vi "DAC Configure FP View.vi"(8 "error in":errorcluster, 11 "DAC TC Temperature in":refnum<class "DAC TC Temperature.lvclass">) -> (0 "error out":errorcluster, 3 "DAC TC Temperature out":refnum<class "DAC TC Temperature.lvclass">)   [LabVIEW 2019, in "DAC.lvlib" / "DAC TC Temperature.lvclass"]
uses:
  DAC TC Temperature.lvclass
  C:/Users/wg/Documents/LV_Projects/test-stand/App/DAC/DAC.lvclass
  Results/Results Method.ctl
  Results/DeepU Results/DeepU Results.lvclass
  DAC.lvclass/DAC.ctl
  DAC TC Temperature.lvclass/DAC TC Temperature.ctl
  Results/Results.lvlib
  DAC.lvclass
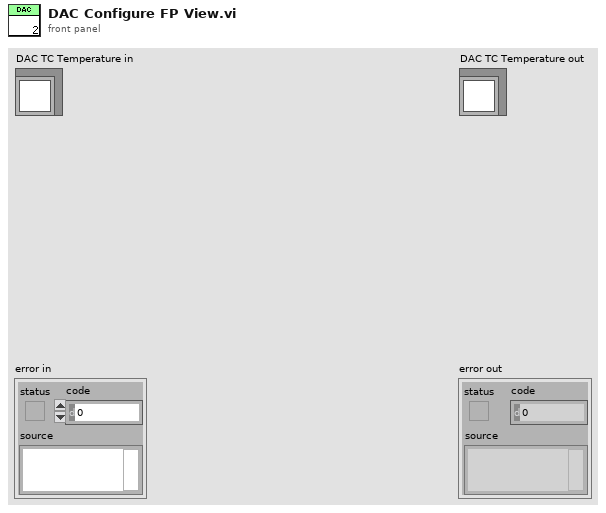
[diagram p1: front panel]
types:
  T1 = typedef "Results.lvlib/Results Method.ctl" = enum16{"Get", "Set"}
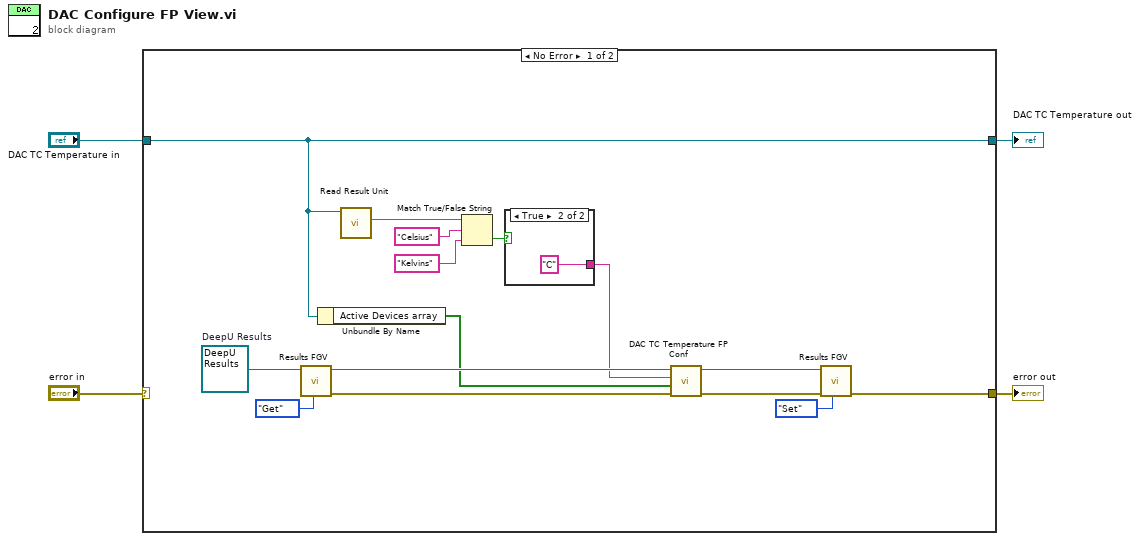
[diagram p0: block diagram]
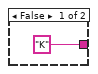
[diagram p2: hidden frame]
diagram:
  n1 = case shown="No Error" "error in" {
    selector: "error in" -> [_ w23]
    tunnel: [w19 w23] -> w1
    tunnel: [w11 w22] -> w2
    tunnel: "DAC TC Temperature in" -> [w11 w22]
    frame No Error {
      w18 = refnum<class "DeepU Results.lvclass"> refnum  # DeepU Results
      n2 = call-dynamic "Results FGV.vi"("Method"=Results_Method."Get", "DeepU Results in"=w18) -> ("error out"=w13:errorcluster, "DeepU Results out"=w15:refnum<class "DeepU Results.lvclass">)  [unwired: 8 in]
      n3 = Unbundle By Name(w11) -> ("Active Devices array"=w10:bool[])
      n4 = call "Read Result Unit.vi"("DAC in"=w11) -> ("Unit"=w6:string)  [unwired: 8 in, 2 out]
      n5 = Match True/False String(2:"Kelvins" ("false string"), 3:"Celsius" ("true string"), 4:w6) -> (0:w7:bool)  [unwired: 1 out]
      n6 = case shown="True" w7 {
        tunnel: ["K" ("false string") "C" ("true string")] -> w5
        frame False {
        }
        frame True {
        }
      }
      n7 = call "DAC TC Temperature FP Conf.vi"("error in (no error)"=w13, "Used TC Temps"=w10, "Result Unit"=w5, "DeepU Results in"=w15) -> ("error out"=w12:errorcluster, "DeepU Results out"=w14:refnum<class "DeepU Results.lvclass">)  [unwired: 6 in]
      n8 = call-dynamic "Results FGV.vi"("Method"=Results_Method."Set", "error in"=w12, "DeepU Results in"=w14) -> ("error out"=w19:errorcluster)  [unwired: 7 in, 1 out]
    }
    frame Error {
    }
  }
  "error out" <- w1
  "DAC TC Temperature out" <- w2
